vi "Read Compressed Image (SubVI).vi"(0 "File REF In":refnum<file>) -> (6 "Frame Number":u64, 8 "TimeStamp":u64, 10 "EOF":bool, 14 "Bit Depth":u8[](array[numeric]), 16 "Minimum":u8[](array[numeric]), 19 "Data":u64[](array[numeric]))   [LabVIEW 2020]
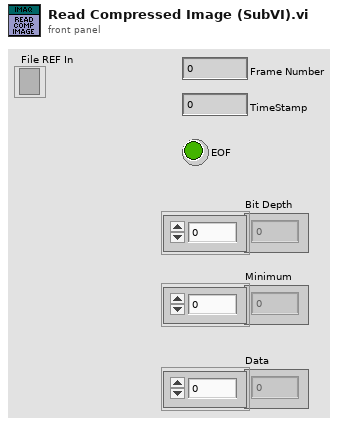
[diagram p1: front panel]
types:
  T1 = enum16{"big-endian, network order", "native, host order", "little-endian"}
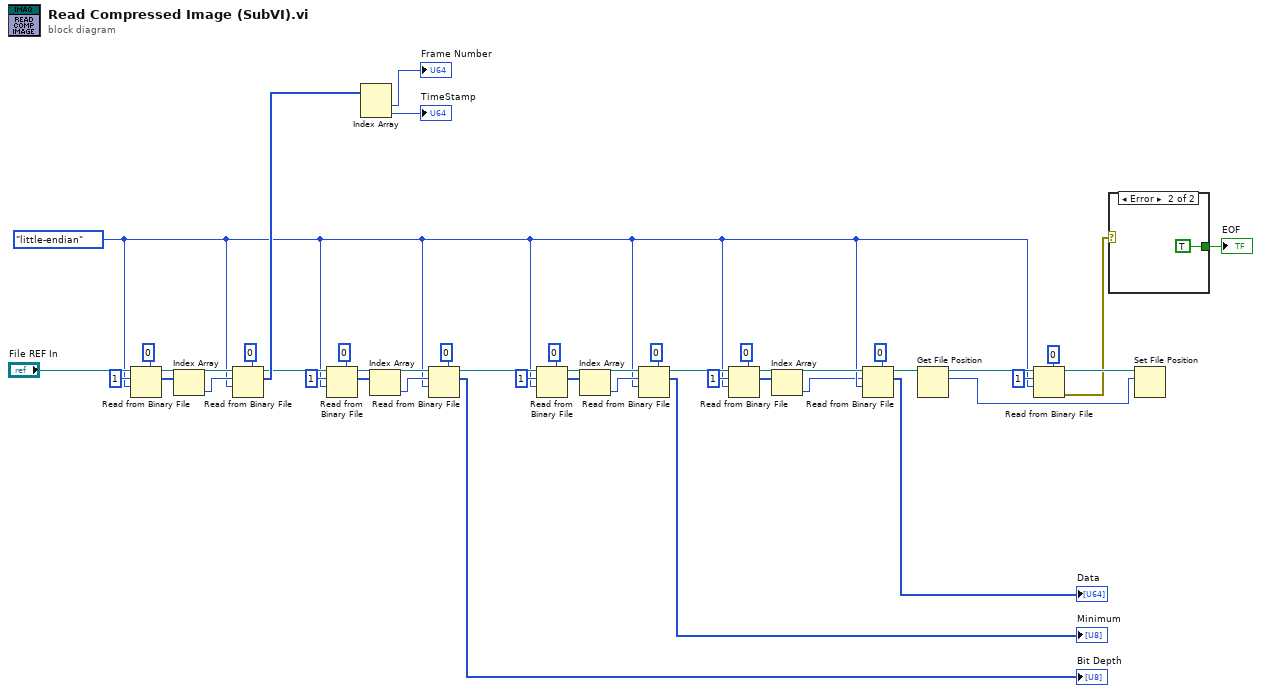
[diagram p0: block diagram]
diagram:
  w2 = T1."little-endian" ("byte order (0:big-endian, network order)")
  n1 = Read from Binary File(5:0 ("count (1)"), 9:w2, 10:1 ("count (1)"), 11:"File REF In") -> (2:w29:i32[], 3:w30:refnum<file>)  [unwired: 2 in, 2 out]
  n2 = Index Array(array=w29) -> (element=w28:i32)  [unwired: 1 in]
  n3 = Read from Binary File(5:u64 0 ("count (1)"), 9:w2, 10:w28, 11:w30) -> (2:w27:u64[], 3:w7:refnum<file>)  [unwired: 2 in, 2 out]
  n4 = Read from Binary File(5:0 ("count (1)"), 9:w2, 10:1 ("count (1)"), 11:w7) -> (2:w25:i32[], 3:w24:refnum<file>)  [unwired: 2 in, 2 out]
  n5 = Index Array(array=w27) -> (element #1=→"Frame Number":u64, element #2=→"TimeStamp":u64)  [unwired: 2 in]
  n6 = Index Array(array=w25) -> (element=w26:i32)  [unwired: 1 in]
  n7 = Read from Binary File(5:u8 0 ("count (1)"), 9:w2, 10:w26, 11:w24) -> (2:→"Bit Depth":u8[], 3:w4:refnum<file>)  [unwired: 2 in, 2 out]
  n8 = Read from Binary File(5:0 ("count (1)"), 9:w2, 10:1 ("count (1)"), 11:w4) -> (2:w15:i32[], 3:w16:refnum<file>)  [unwired: 2 in, 2 out]
  n9 = Index Array(array=w15) -> (element=w14:i32)  [unwired: 1 in]
  n10 = Read from Binary File(5:u8 0 ("count (1)"), 9:w2, 10:w14, 11:w16) -> (2:→"Minimum":u8[], 3:w5:refnum<file>)  [unwired: 2 in, 2 out]
  n11 = Read from Binary File(5:0 ("count (1)"), 9:w2, 10:1 ("count (1)"), 11:w5) -> (2:w12:i32[], 3:w11:refnum<file>)  [unwired: 2 in, 2 out]
  n12 = Index Array(array=w12) -> (element=w1:i32)  [unwired: 1 in]
  n13 = Read from Binary File(5:u64 0 ("count (1)"), 9:w2, 10:w1, 11:w11) -> (2:→"Data":u64[], 3:w6:refnum<file>)  [unwired: 2 in, 2 out]
  n14 = Get File Position(7:w6) -> (2:w32:i64, 3:w33:refnum<file>)  [unwired: 1 in, 1 out]
  n15 = Read from Binary File(5:u8 0, 9:w2, 10:1 ("count (1)"), 11:w33) -> (0:w36:errorcluster, 3:w38:refnum<file>)  [unwired: 2 in, 2 out]
  n16 = case shown="Error" w36 {
    tunnel: [_ TRUE] -> w35
    frame No Error {
    }
    frame Error {
    }
  }
  "EOF" <- w35
  n17 = Set File Position(offset (in bytes) (0)=w32, refnum=w38) -> ()  [unwired: 2 in, 2 out]
